vi "LibXML_GetAttrValueByName.vi"(8 "error in":errorcluster, 10 "attribute":string, 11 "node":u32) -> (0 "error out":errorcluster, 1 "Found":bool, 3 "lvstring":string)   [LabVIEW 2019, in "Tools.lvlib" / "LibXML.lvlib"]
doc: "Get the attribute of a node by attribute name."
uses:
  LibXML.lvlib
  Error Cluster From Error Code_subroutine.vi
  <vilib>/Utility/error.llb/Trim Whitespace.vi
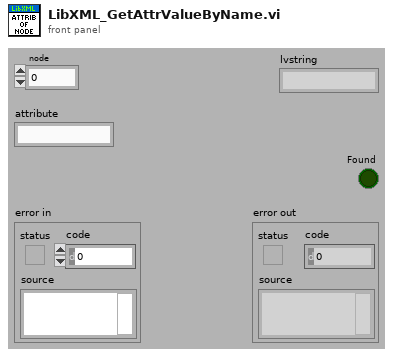
[diagram p1: front panel]
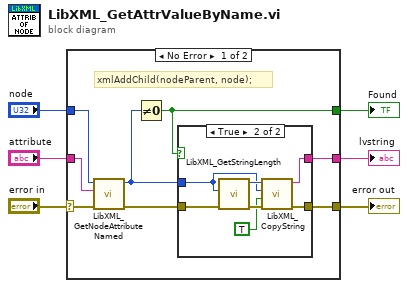
[diagram p0: block diagram]
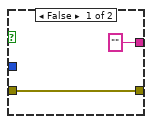
[diagram p2: hidden frame]
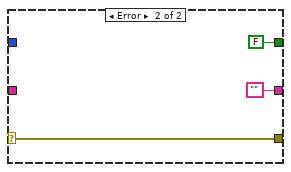
[diagram p3: hidden frame]
diagram:
  n1 = case shown="No Error" "error in" {
    selector: "error in" -> [w13 w26]
    tunnel: [w12 w26] -> w5
    tunnel: [w10 FALSE] -> w4
    tunnel: [w9 ""] -> w3
    tunnel: "node" -> [w8 _]
    tunnel: "attribute" -> [w7 _]
    frame No Error {
      # "xmlAddChild(nodeParent, node);"
      n2 = call "LibXML_GetNodeAttributeNamed.vi"("error in"=w13, "attribute name"=w7, "node"=w8) -> ("error out"=w14:errorcluster, "string pointer"=w11:u32)  [unwired: 7 in]
      n3 = Not Equal To 0?(x=w11) -> (x != 0?=w10:bool)
      n4 = case shown="True" w10 {
        tunnel: ["" ("lvstring") w23] -> w9
        tunnel: w14 -> [w16 w22]
        tunnel: w11 -> [_ w19]
        tunnel: [w16 w17] -> w12
        frame False {
        }
        frame True {
          n5 = call "LibXML_GetStringLength.vi"("error in"=w22, "string pointer"=w19) -> ("error out"=w21:errorcluster, "string length"=w20:i32)  [unwired: 4 in]
          n6 = call "LibXML_CopyString.vi"("error in"=w21, "free pointer?"=TRUE, "string pointer"=w19, "length"=w20) -> ("error out"=w17:errorcluster, "lvstring"=w23:string)  [unwired: 6 in]
        }
      }
    }
    frame Error {
    }
  }
  "error out" <- w5
  "Found" <- w4
  "lvstring" <- w3
